vi "Shutdown Boiler.vi"(7 "MHL Queue in":refnum<queue>, 8 "error in":errorcluster, 9 "UI Data in":T1, 10 "Handshake Notifier in":refnum<notifier>, 11 "Boiler Queue in":refnum<queue>) -> (0 "error out":errorcluster, 1 "UI Data out":T1, 2 "Handshake Notifier out":refnum<notifier>, 3 "Boiler Queue out":refnum<queue>, 5 "MHL Queue out":refnum<queue>)   [LabVIEW 2022 SP3, in "Controller.lvlib"]
doc: "Shut down the boiler."
uses:
  Controller.lvlib
  Course Project/support/Message Queue/Message Cluster.ctl
  controls/MHL UI Data.ctl
  controls/MHL Status.ctl
  Support VIs/Boiler System Globals.vi
  Course Project/support/Message Queue/Message Queue.lvlib
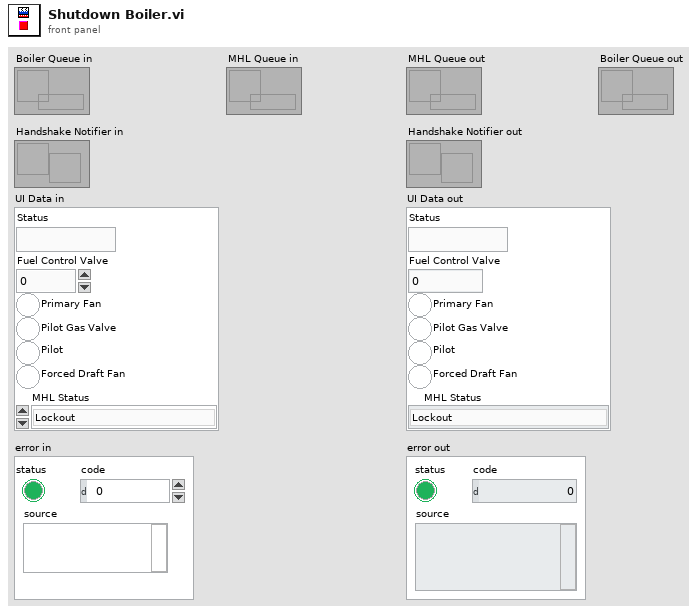
[diagram p1: front panel]
types:
  T1 = typedef "MHL UI Data.ctl" = cluster{"Status":string, "Fuel Control Valve":u32, "Primary Fan":bool, "Pilot Gas Valve":bool, "Pilot":bool, "Forced Draft Fan":bool, "MHL Status":T2}
  T2 = typedef "MHL Status.ctl" = enum16{"Lockout", "Ready", "Pre-Purge", "Pre-Purge Complete", "Pilot On", "Boiler Running", "Shutdown", "Purge"}
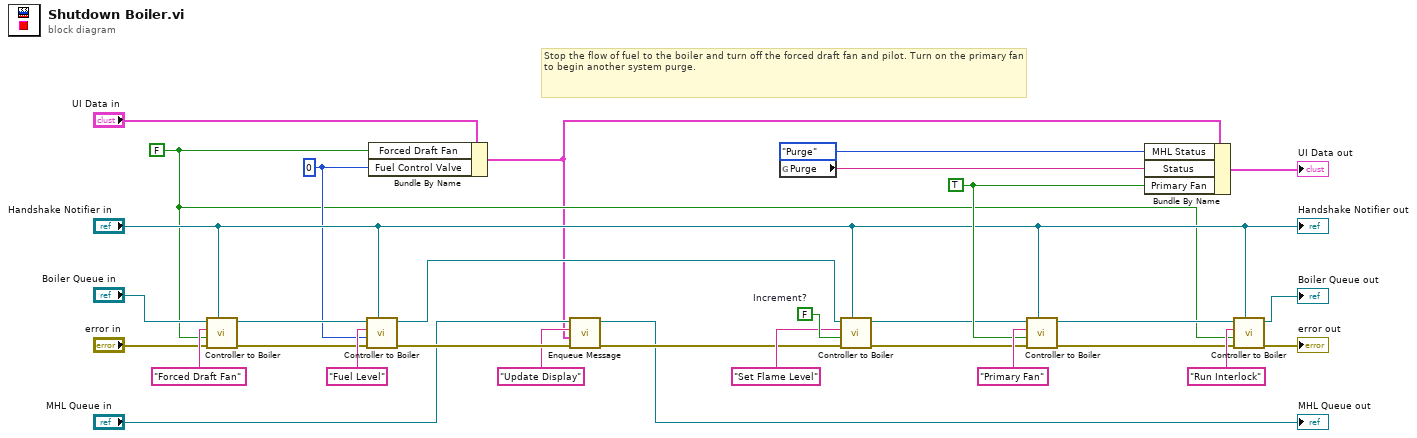
[diagram p0: block diagram]
diagram:
  w5 = u32 0 ("Fuel Control Valve Position Value")
  w4 = FALSE ("Fuel Valve")
  w23 = TRUE ("Primary Fan")
  w29 = FALSE  # Increment?
  # "Stop the flow of fuel to the boiler and turn off the forced draft fan and pilot. Turn on the primary fan to begin another system purge."
  n1 = call "Controller to Boiler.vi"("Notifier"="Handshake Notifier in", "error in"="error in", "Message Data"=w4, "Message"="Forced Draft Fan", "Boiler Queue in"="Boiler Queue in") -> ("error out"=w15:errorcluster, "Queue out"=w12:refnum<queue>)  [unwired: 4 in, 1 out]
  n2 = call "Controller to Boiler.vi"("Notifier"="Handshake Notifier in", "error in"=w15, "Message Data"=w5, "Message"="Fuel Level", "Boiler Queue in"=w12) -> ("error out"=w14:errorcluster, "Queue out"=w13:refnum<queue>)  [unwired: 4 in, 1 out]
  n3 = Bundle By Name(cluster="UI Data in", "Forced Draft Fan"=w4, "Fuel Control Valve"=w5) -> (w3:T1)
  n4 = call "Enqueue Message.vi"("error in"=w14, "Message Data"=w3, "Message"="Update Display", "Message Queue"="MHL Queue in") -> ("error out"=w9:errorcluster, "dup Message Queue"=→"MHL Queue out":refnum<queue>)  [unwired: 6 in]
  n5 = global read "Boiler System Globals.vi" "Purge"() -> (w21:string)
  n6 = call "Controller to Boiler.vi"("Notifier"="Handshake Notifier in", "error in"=w9, "Message Data"=w29, "Message"="Set Flame Level", "Boiler Queue in"=w13) -> ("error out"=w11:errorcluster, "Queue out"=w10:refnum<queue>)  [unwired: 4 in, 1 out]
  n7 = call "Controller to Boiler.vi"("Notifier"="Handshake Notifier in", "error in"=w11, "Message Data"=w23, "Message"="Primary Fan", "Boiler Queue in"=w10) -> ("error out"=w25:errorcluster, "Queue out"=w24:refnum<queue>)  [unwired: 4 in, 1 out]
  n8 = Bundle By Name(cluster=w3, "MHL Status"=MHL_Status."Purge", "Status"=w21, "Primary Fan"=w23) -> (→"UI Data out":T1)
  n9 = call "Controller to Boiler.vi"("Notifier"="Handshake Notifier in", "error in"=w25, "Message Data"=w4, "Message"="Run Interlock", "Boiler Queue in"=w24) -> ("error out"=→"error out":errorcluster, "Queue out"=→"Boiler Queue out":refnum<queue>)  [unwired: 4 in, 1 out]
  "Handshake Notifier out" <- "Handshake Notifier in"
